vi "ForceSetpointHandler.vi"(2 "Force Setpoints":i32[](array[numeric])) -> (0 "Force Setpoint":i32)   [LabVIEW 2014]
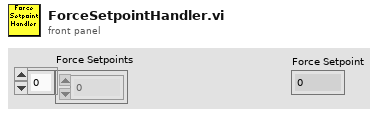
[diagram p1: front panel]
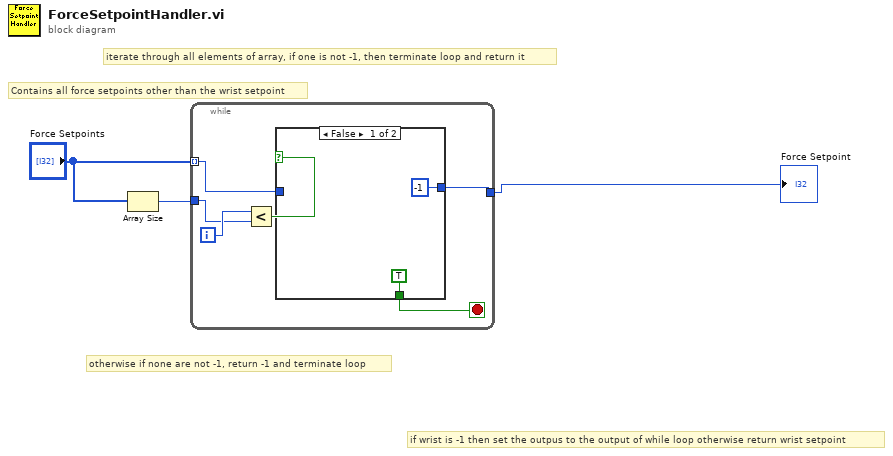
[diagram p0: block diagram]
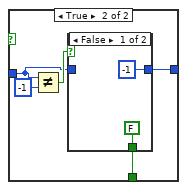
[diagram p2: hidden frame]
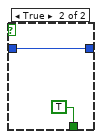
[diagram p3: hidden frame]
diagram:
  # "if wrist is -1 then set the outpus to the output of while loop otherwise return wrist setpoint"
  # "otherwise if none are not -1, return -1 and terminate loop"
  # "iterate through all elements of array, if one is not -1, then terminate loop and return it"
  # "Contains all force setpoints other than the wrist setpoint"
  n1 = Array Size(array="Force Setpoints") -> (size(s)=w2:i32)
  n2 = while {
    tunnel: "Force Setpoints" -> [w6] mode=indexing
    tunnel: w2 -> [w8]
    tunnel: [w4] -> w1
    i -> [w9]
    stop <- w5 stop-if-true
    n3 = Less?(x=w9, y=w8) -> (x < y?=w7:bool)
    n4 = case shown="False" w7 {
      tunnel: w6 -> [_ w13]
      tunnel: [TRUE w14] -> w5
      tunnel: [-1 ("Numeric") w12] -> w4
      frame False {
      }
      frame True {
        n5 = Not Equal?(x=w13, y=-1) -> (x != y?=w15:bool)
        n6 = case shown="False" w15 {
          tunnel: [FALSE TRUE] -> w14
          tunnel: w13 -> [_ w19]
          tunnel: [-1 ("Numeric") w19] -> w12
          frame False {
          }
          frame True {
          }
        }
      }
    }
  }
  "Force Setpoint" <- w1
